vi "Warning_C13.vi"(7 "Warning in":string) -> ()   [LabVIEW 2020]
doc: "This VI Dispalys the Error Popup Window with Error Message given as input to it."
panel:
  in  "OK":bool caption="Boolean"
  out "Warning":string
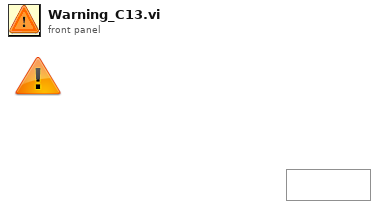
[diagram p1: front panel]
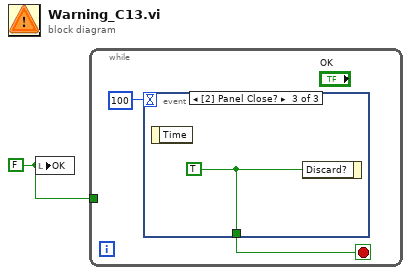
[diagram p0: block diagram]
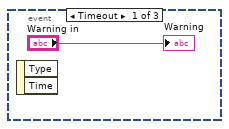
[diagram p2: hidden frame]
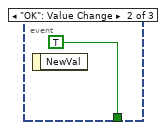
[diagram p3: hidden frame]
diagram:
  w1 = FALSE ("OK")
  n1 = local write "OK"(w1) -> ()
  n2 = while {
    tunnel: w1 -> [_]
    stop <- w3 stop-if-true
    n3 = event shown="[2] Panel Close?" {
      selector: _ -> [_ _ _]
      dyn-events: _ -> [_ _ _]
      timeout: 100 -> [_ _ _]
      tunnel: [_ TRUE ("NewVal") w6] -> w3
      event Timeout {
        n4 = event-data() -> ()  [unwired: 1 in, 2 out]
        "Warning" <- "Warning in"
      }
      event "OK": Value Change {
        n5 = event-data() -> ()  [unwired: 1 in, 1 out]
      }
      event Panel Close? {
        w6 = TRUE ("Discard?")
        n6 = event-data() -> ()  [unwired: 1 in, 1 out]
        n7 = event-data("Discard?"=w6) -> ()  [unwired: 1 in, 1 out]
      }
    }
  }
